vi "Get Size.vi"(11 "Map in":refnum<class "Map.lvclass">) -> (2 "Size":i32, 3 "Map out":refnum<class "Map.lvclass">)   [LabVIEW 2020, in "SquareBattle.lvlib" / "Map.lvclass"]
uses:
  Map.lvclass
  Map.lvclass/Map.ctl
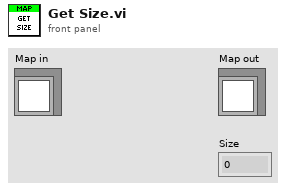
[diagram p1: front panel]
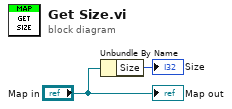
[diagram p0: block diagram]
diagram:
  n1 = Unbundle By Name("Map in") -> ("Size"=→"Size":i32)
  "Map out" <- "Map in"
